vi "Temperature Limit.vi"() -> ()   [LabVIEW 2015]
doc: "This VI simulates the acquisition of temperature, graphs the temperature, and notifies the user if the temperature is over the limit."
panel:
  in  "Start":bool
  in  "Delta t (ms)":i32(slide)=400 scale=50.0..500.0
  in  "Stop":bool
  in  "High Limit":dbl=28.0 format="%.2f"
  out "Temperature":cluster{"Temperature":dbl, "High Limit":dbl}(graph)={"Temperature"=85.88749999999999, "High Limit"=80.0}
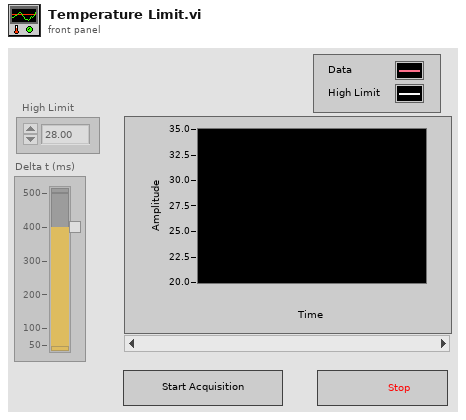
[diagram p1: front panel]
types:
  T1 = enum8{"Enabled", "Disabled", "Disabled and Grayed Out"}
  T2 = cluster{"Temperature Value":dbl, "High Limit":dbl}
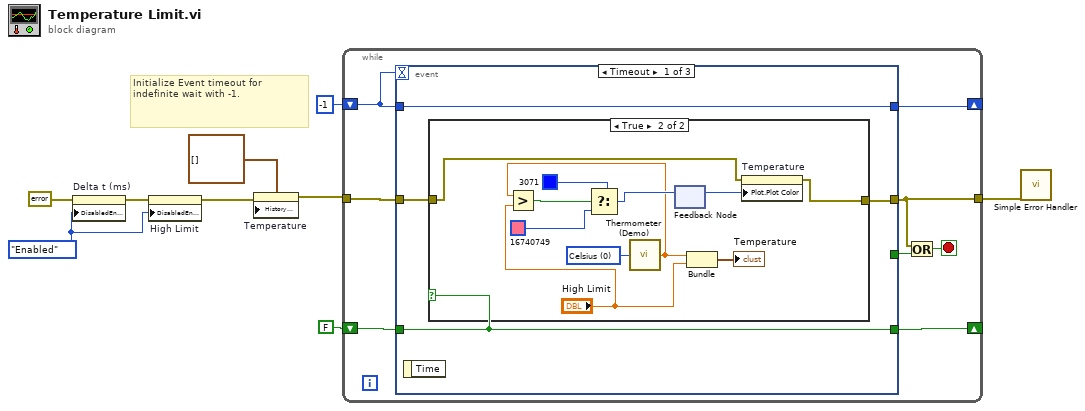
[diagram p0: block diagram]
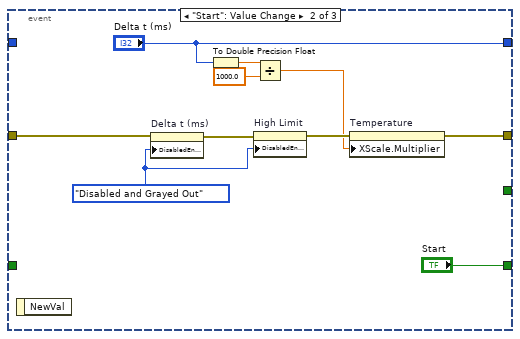
[diagram p3: hidden frame]
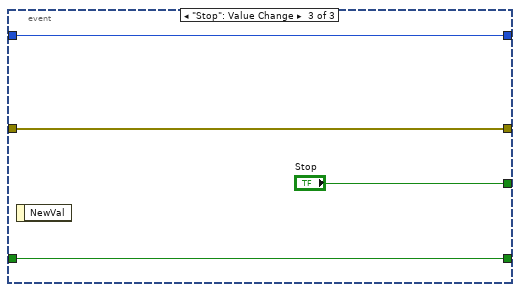
[diagram p4: hidden frame]
diagram:
  w4 = T1."Enabled" ("Disabled")
  # "Initialize Event timeout for indefinite wait with -1."
  n1 = property on="Delta t (ms)" class="Slide (strict)"(error in=errorcluster {"status"=FALSE, "code"=0, "source"=""} ("error out"), "DisabledEnum"=w4) -> (error out=w5:errorcluster)  [unwired: 1 in, 1 out]
  n2 = property on="High Limit" class="DigNum (strict)"(error in=w5, "DisabledEnum"=w4) -> (error out=w3:errorcluster)  [unwired: 1 in, 1 out]
  n3 = property on="Temperature" class="WFChart (strict)"(error in=w3, "History Data"=cluster{"Temperature":dbl, "High Limit":dbl}[] []) -> (error out=w2:errorcluster)  [unwired: 1 in, 1 out]
  n4 = while {
    tunnel: w2 -> [w17]
    tunnel: [w15] -> w8
    shift-right: [w13] -> _
    shift-left: FALSE ("Start") -> [w12]
    shift-right: [w11] -> _
    shift-left: -1 ("Delta t (ms)") -> [w10]
    stop <- w16 stop-if-true
    n5 = event shown="[0] Timeout" {
      selector: _ -> [_ _ _]
      dyn-events: _ -> [_ _ _]
      timeout: w10 -> [_ _ _]
      tunnel: [_ _ "Stop"] -> w14
      tunnel: w17 -> [w19 w42 w46]
      tunnel: [w18 w39 w46] -> w15
      tunnel: [w20 "Start" w45] -> w13
      tunnel: w12 -> [w20 _ w45]
      tunnel: [w21 "Delta t (ms)" w44] -> w11
      tunnel: w10 -> [w21 _ w44]
      event Timeout {
        n6 = event-data() -> ()  [unwired: 1 in, 1 out]
        n7 = case shown="True" w20 {
          tunnel: w19 -> [w22 w24]
          tunnel: [w22 w23] -> w18
          frame False {
          }
          frame True {
            w32 = u16 0 items=["Celsius", "Fahrenheit"] ("Units (0: Celsius)")
            n8 = call "Thermometer (Demo).vi"("Units (0: Celsius)"=w32) -> ("Temperature Value"=w26:dbl)
            n9 = Greater?(x=w26, y="High Limit") -> (0:w31:bool)
            n10 = Select(t=u32 3071, s=w31, f=u32 16740749) -> (s? t:f=w29:u32)
            n11 = feedback #1() -> (w25:u32)  [unwired: 1 in]
            n12 = feedback-in #1(w29) -> ()
            n13 = Bundle("Temperature Value"=w26, "High Limit"="High Limit") -> (→"Temperature":T2)  [unwired: 1 in]
            n14 = property on="Temperature" class="WFChart (strict)"(error in=w24, "Plot.Plot Color"=w25) -> (error out=w23:errorcluster)  [unwired: 1 in, 1 out]
          }
        }
      }
      event "Start": Value Change {
        w38 = T1."Disabled and Grayed Out" ("Disabled")
        n15 = event-data() -> ()  [unwired: 1 in, 1 out]
        n16 = property on="Delta t (ms)" class="Slide (strict)"(error in=w42, "DisabledEnum"=w38) -> (error out=w41:errorcluster)  [unwired: 1 in, 1 out]
        n17 = To Double Precision Float(number="Delta t (ms)") -> (double precision float=w36:dbl)
        n18 = property on="High Limit" class="DigNum (strict)"(error in=w41, "DisabledEnum"=w38) -> (error out=w40:errorcluster)  [unwired: 1 in, 1 out]
        n19 = Divide(x=w36, y=1000.0) -> (x/y=w34:dbl)
        n20 = property on="Temperature" class="WFChart (strict)"(error in=w40, "XScale.Multiplier"=w34) -> (error out=w39:errorcluster)  [unwired: 1 in, 1 out]
      }
      event "Stop": Value Change {
        n21 = event-data() -> ()  [unwired: 1 in, 1 out]
      }
    }
    n22 = Or(x=w15, y=w14) -> (x .or. y?=w16:bool)
  }
  n23 = call <vilib>:"Simple Error Handler.vi"("error in (no error)"=w8) -> ()  [unwired: 4 in, 5 out]
